vi "Reshape 3D to 2D data.vi"(0 "Parameters In (3D)":cdb[][][](array[numeric]) format="%.3f", 11 "Error In":errorcluster) -> (4 "Parameters Out (2D)":cdb[][](array[numeric]) format="%.3f", 15 "Error Out":errorcluster)   [LabVIEW 2023, in "NI_HFNetworkAnalysis.lvlib"]
doc: "Transforms a 3D array of network parameters into a 2D array.\n\nInput 3D array pages are assumed as\n<b>((x11,x12,x13,...),\n (x21,x22,x23,...),\n (x31,x32,x33,...),\n ...)</b>\nand resulting 2D array rows are defined as\n<b>(x11,x12,x13,...,x21,x22,x23,...,x31,x32,x33,...)</b>"
uses:
  NI_HFNetworkAnalysis.lvlib
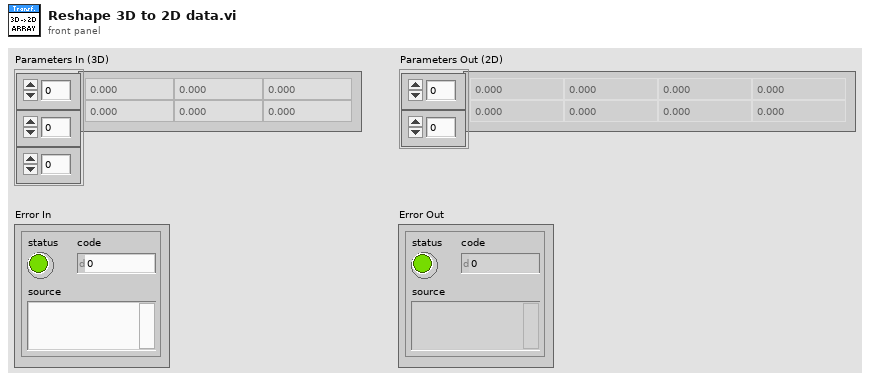
[diagram p1: front panel]
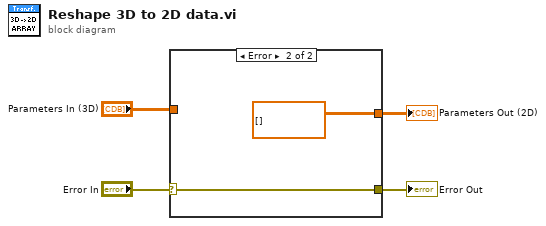
[diagram p0: block diagram]
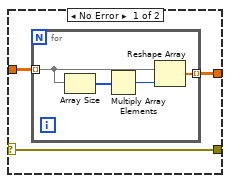
[diagram p2: hidden frame]
diagram:
  n1 = case shown="Error" "Error In" {
    selector: "Error In" -> [w5 w12]
    tunnel: "Parameters In (3D)" -> [w7 _]
    tunnel: [w6 cdb[][] []] -> w3
    tunnel: [w5 w12] -> w1
    frame No Error {
      n2 = for {
        tunnel: w7 -> [w8] mode=indexing
        tunnel: [w9] -> w6 mode=indexing
        n3 = Array Size(array=w8) -> (size(s)=w11:i32[])
        n4 = Multiply Array Elements(1:w11) -> (0:w10:i32)
        n5 = Reshape Array(w8, w10) -> (w9:cdb[])
      }
    }
    frame Error {
    }
  }
  "Parameters Out (2D)" <- w3
  "Error Out" <- w1
